vi "Set Or Get Visible Items.vi"(8 "error in (no error)":errorcluster caption="错误输入（无错误）", 9 "Mode":T2, 10 "Disp In":T1, 11 "Table Ref In":refnum<vi>) -> (0 "error out":errorcluster caption="错误输出", 2 "Disp Out":T1, 3 "Table Ref Out":refnum<vi>)   [LabVIEW 2012, in "Table Tool.lvlib"]
uses:
  Table Tool.lvlib
  GetOrSet.ctl
  Disp.ctl
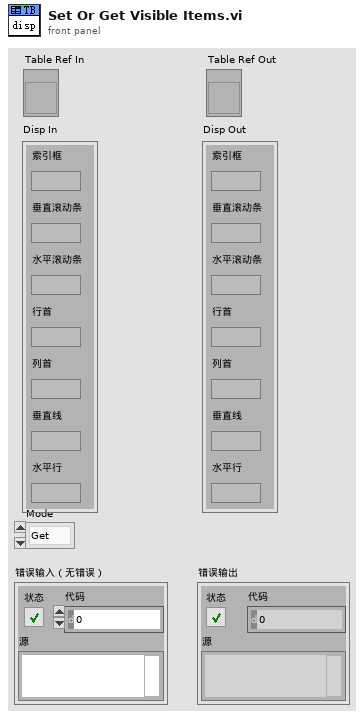
[diagram p1: front panel]
types:
  T1 = typedef "Table Tool.lvlib/Disp.ctl" = cluster{"索引框":bool, "垂直滚动条":bool, "水平滚动条":bool, "行首":bool, "列首":bool, "垂直线":bool, "水平行":bool}
  T2 = typedef "Table Tool.lvlib/GetOrSet.ctl" = enum16{"Get", "Set"}
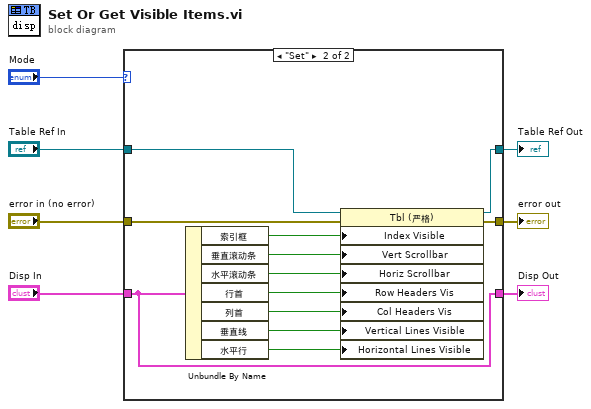
[diagram p0: block diagram]
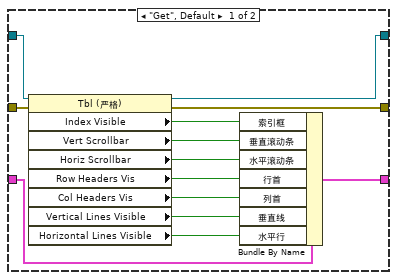
[diagram p2: hidden frame]
diagram:
  n1 = case shown="\"Set\"" "Mode" {
    tunnel: "Table Ref In" -> [w19 w31]
    tunnel: "error in (no error)" -> [w20 w32]
    tunnel: [w17 w29] -> w4
    tunnel: [w18 w30] -> w3
    tunnel: [w8 w21] -> w1
    tunnel: "Disp In" -> [w16 w21]
    frame "Get", Default {
      n2 = property class="Tbl (严格)"(reference=w19, error in=w20) -> (reference out=w18:refnum<vi>, error out=w17:errorcluster, "Index Visible"=w15:bool, "Vert Scrollbar"=w14:bool, "Horiz Scrollbar"=w13:bool, "Row Headers Vis"=w12:bool, "Col Headers Vis"=w11:bool, "Vertical Lines Visible"=w10:bool, "Horizontal Lines Visible"=w9:bool)
      n3 = Bundle By Name(cluster=w16, "索引框"=w15, "垂直滚动条"=w14, "水平滚动条"=w13, "行首"=w12, "列首"=w11, "垂直线"=w10, "水平行"=w9) -> (w8:T1)
    }
    frame "Set" {
      n4 = Unbundle By Name(w21) -> ("索引框"=w28:bool, "垂直滚动条"=w27:bool, "水平滚动条"=w26:bool, "行首"=w25:bool, "列首"=w24:bool, "垂直线"=w23:bool, "水平行"=w22:bool)
      n5 = property class="Tbl (严格)"(reference=w31, error in=w32, "Index Visible"=w28, "Vert Scrollbar"=w27, "Horiz Scrollbar"=w26, "Row Headers Vis"=w25, "Col Headers Vis"=w24, "Vertical Lines Visible"=w23, "Horizontal Lines Visible"=w22) -> (reference out=w30:refnum<vi>, error out=w29:errorcluster)
    }
  }
  "Table Ref Out" <- w3
  "error out" <- w4
  "Disp Out" <- w1
